vi "PrepareIESourceCore.vi"(8 "error in (no error)":errorcluster) -> (0 "error out":errorcluster)   [LabVIEW 2021]
uses:
  <userlib>/_OpenG.lib/lvzip/lvzip.llb/ZLIB Open ZIP Mode__ogtk.ctl
  <userlib>/_OpenG.lib/file/file.llb/Convert File Extension (Path)__ogtk.vi
  <userlib>/_OpenG.lib/lvzip/lvzip.llb/subVI/ZLIB Compress Directory (Path)__ogtk.vi
  <vilib>/Utility/config.llb/Write Key (String).vi
  <userlib>/_OpenG.lib/file/file.llb/openg_file.lvlib
  <vilib>/Utility/config.llb/NI_LVConfig.lvlib
panel:
  # "Prepare"
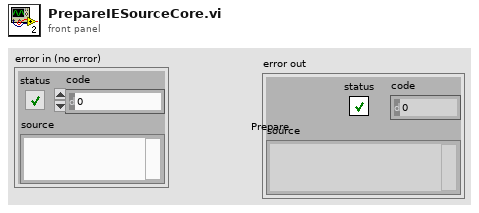
[diagram p1: front panel]
types:
  T1 = typedef "ZLIB Open ZIP Mode__ogtk.ctl" = enum16{"create new", "append to end", "append to archive"}
  T2 = typedef "NI_LVConfig.lvlib/Config Data RefNum.ctl" = refnum<k1>
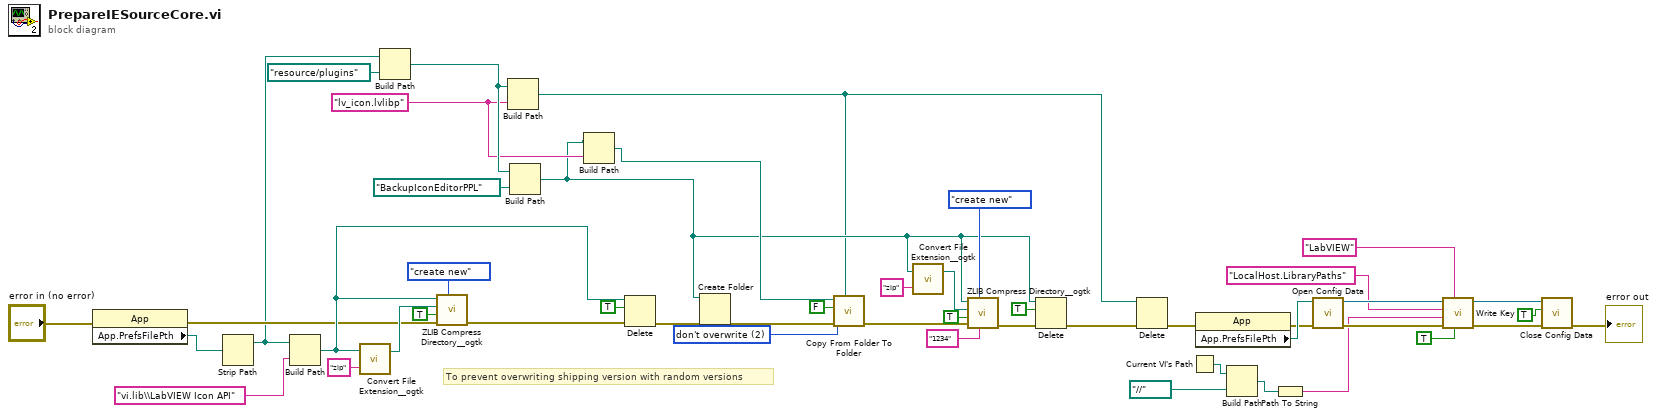
[diagram p0: block diagram]
diagram:
  w27 = u16 2 items=["overwrite", "ask first", "don't overwrite"] ("overwrite")
  w24 = "lv_icon.lvlibp" ("name")
  # "To prevent overwriting shipping version with random versions"
  n1 = property class="App"(error in="error in (no error)") -> (error out=w40:errorcluster, "App.PrefsFilePth"=w48:path)  [unwired: 1 in, 1 out]
  n2 = Strip Path(path=w48) -> (stripped path=w37:path)  [unwired: 1 out]
  n3 = Build Path(base path=w37, name or relative path="vi.lib\\LabVIEW Icon API" ("name")) -> (appended path=w42:path)
  n4 = call-poly <userlib>:"Convert File Extension__ogtk.vi"("new ending (none)"="zip", "file name"=w42) -> ("new filename"=w43:path)  [unwired: 1 out]
  n5 = Build Path(base path=w37, name or relative path=path "resource/plugins") -> (appended path=w26:path)
  n6 = call-poly <userlib>:"ZLIB Compress Directory__ogtk.vi"("append (create new)"=ZLIB_Open_ZIP_Mode__ogtk."create new", "error in (no error)"=w40, "include subdirectories (F)"=TRUE, "archive name (root directory with .zip ending)"=w43, "root directory (file dialog)"=w42) -> ("error out"=w38:errorcluster)  [unwired: 4 in, 2 out]
  n7 = Build Path(base path=w26, name or relative path=w24) -> (appended path=w18:path)
  n8 = Build Path(base path=w26, name or relative path=path "BackupIconEditorPPL") -> (appended path=w20:path)
  n9 = Build Path(base path=w20, name or relative path=w24) -> (appended path=w23:path)
  n10 = Delete(path (use dialog)=w42, entire hierarchy (F)=TRUE, error in=w38) -> (error out=w35:errorcluster)  [unwired: 2 in, 2 out]
  n11 = Create Folder(path (use dialog)=w20, error in=w35) -> (error out=w33:errorcluster)  [unwired: 1 in, 2 out]
  n12 = call <vilib>:"Copy From Folder To Folder.vi"("source"=w18, "error in (no error)"=w33, "overwrite"=w27, "remove original (F)"=FALSE, "destination"=w23) -> ("error out"=w31:errorcluster)  [unwired: 5 in, 1 out]
  n13 = call-poly <userlib>:"Convert File Extension__ogtk.vi"("new ending (none)"="zip", "file name"=w20) -> ("new filename"=w30:path)  [unwired: 1 out]
  n14 = call-poly <userlib>:"ZLIB Compress Directory__ogtk.vi"("password (none)"="1234", "append (create new)"=ZLIB_Open_ZIP_Mode__ogtk."create new", "error in (no error)"=w31, "include subdirectories (F)"=TRUE, "archive name (root directory with .zip ending)"=w30, "root directory (file dialog)"=w20) -> ("error out"=w22:errorcluster)  [unwired: 3 in, 2 out]
  n15 = Delete(path (use dialog)=w20, entire hierarchy (F)=TRUE, error in=w22) -> (error out=w21:errorcluster)  [unwired: 2 in, 2 out]
  n16 = Delete(path (use dialog)=w18, error in=w21) -> (error out=w5:errorcluster)  [unwired: 3 in, 2 out]
  n17 = Current VI's Path() -> (path=w15:path)
  n18 = property class="App"(error in=w5) -> (error out=w13:errorcluster, "App.PrefsFilePth"=w14:path)  [unwired: 1 in, 1 out]
  n19 = Build Path(base path=w15, name or relative path=path "../../..") -> (appended path=w3:path)
  n20 = Path To String(path=w3) -> (string=w2:string)
  n21 = call <vilib>:"Open Config Data.vi"("error in (no error)"=w13, "configuration file path"=w14) -> ("error out"=w11:errorcluster, "refnum"=w10:T2)  [unwired: 7 in, 1 out]
  n22 = call-poly <vilib>:"Write Key.vi"("write raw string? (F)"=TRUE, "section"="LabVIEW", "error in (no error)"=w11, "value"=w2, "key"="LocalHost.LibraryPaths", "refnum"=w10) -> ("error out"=w6:errorcluster, "refnum out"=w7:T2)  [unwired: 3 in, 1 out]
  n23 = call <vilib>:"Close Config Data.vi"("error in (no error)"=w6, "write file if changed (T)"=TRUE, "refnum"=w7) -> ("error out"=→"error out":errorcluster)  [unwired: 7 in, 1 out]
